vi "oa_Build Spectral Info for Order Magnitude and Phase (N Channels).vi"(0 "channel info":T8[](array[typedef]) {"channel info"."pregain" format="%.2f"; "channel info"."weighting filter" items=["Linear", "A-weighting", "B-weighting", "C-weighting", "ITU-R 468-4", "Dolby", "CCITT", "C-message", "Wb", "Wc", "Wd", "We", "Wf", "Wh", "Wj", "Wk", "Wm", "AES17 20 kHz lowpass", "AES17 40 kHz lowpass", "AES17 20 kHz highpass", "AES17 40 kHz highpass"]; "channel info"."dB reference" format="%^.1e"; "channel info"."engineering units" items=["custom..."=0, "V"=1, "A"=21, "C"=30, "pC"=31, "s"=32, "-"=29, "Pa"=2, "N"=20, "g"=3, "m/s^2"=4, "m/s"=5, "m"=6, "mm/s"=12, "mm"=13, "micron/s"=14, "micron"=15, "in/s^2"=7, "in/s"=8, "in"=9, "mil/s"=10, "mil"=11, "rad/s^2"=16, "rad/s"=17, "rad"=18, "deg/s^2"=26, "deg/s"=27, "deg"=28, "RPM"=22, "cycle/s^2"=23, "Hz"=24, "cycle"=25, "strain"=19]; "channel info"."sensor sensitivity" format="%#_5f"}, 1 "reset? (T)":bool=TRUE, 5 "X axis selection":u16(ring)=2 items=["Time", "Revolution", "RPM"], 7 "unit labels":string[](array[string]), 9 "orders to compute":dbl[](array[numeric]) format="%.2f", 11 "error in (no error)":errorcluster, 12 "view":T1={"dB on? (T)"=FALSE, "unwrap phase? (T)"=TRUE, "unit in degree? (T)"=TRUE}) -> (4 "spectrum info":T2[](array[typedef]) {"x-axis units" items=["Time (s)"=0, "Frequency-CB (Hz)"=1, "Frequency-CPB (Hz)"=1248, "Frequency-Arbitrary (Hz)"=2357, "Quefrency (s)"=2, "Revolutions (rev)"=3, "Order"=4, "Speed (RPM)"=11, "Speed (rad/s)"=21, "Index"=65535]; "weighting filter" items=["Linear", "A-weighting", "B-weighting", "C-weighting", "ITU-R 468-4", "Dolby", "CCITT", "C-message", "Wb", "Wc", "Wd", "We", "Wf", "Wh", "Wj", "Wk", "Wm", "AES17 20 kHz lowpass", "AES17 40 kHz lowpass", "AES17 20 kHz highpass", "AES17 40 kHz highpass"]; "dB reference [EU]" format="%.2f"; "engineering units" items=["custom..."=0, "V"=1, "A"=21, "C"=30, "pC"=31, "s"=32, "-"=29, "Pa"=2, "N"=20, "g"=3, "m/s^2"=4, "m/s"=5, "m"=6, "mm/s"=12, "mm"=13, "micron/s"=14, "micron"=15, "in/s^2"=7, "in/s"=8, "in"=9, "mil/s"=10, "mil"=11, "rad/s^2"=16, "rad/s"=17, "rad"=18, "deg/s^2"=26, "deg/s"=27, "deg"=28, "RPM"=22, "cycle/s^2"=23, "Hz"=24, "cycle"=25, "strain"=19]; "spectral info"."window" items=["None "=0, "Hanning"=1, "Hamming"=2, "Blackman-Harris"=3, "Exact Blackman"=4, "Blackman"=5, "Flat Top"=6, "4 Term B-Harris "=7, "7 Term B-Harris"=8, "Low Sidelobe"=9, "Force - Exponential"=10, "Gaussian"=62]}, 15 "error out":errorcluster)   [LabVIEW 2017, in "SoundVib_Resampling.lvlib"]
uses:
  <vilib>/addons/Sound and Vibration/Order Analysis/Resample Order Tracking/SoundVib_Resampling.lvlib
  <vilib>/addons/_NISVFA/_Shared subVIs/Controls/svc_Resampled Channel Info.ctl
  <vilib>/addons/_NISVFA/_Shared subVIs/Controls/svc_Channel Info.ctl
  <vilib>/addons/_NISVFA/_Shared subVIs/Controls/svc_Engineering Units Text Ring.ctl
  <vilib>/addons/_NISVFA/_Shared subVIs/Controls/svc_Weighting Filter Text Ring.ctl
  <vilib>/addons/_NISVFA/_Shared subVIs/Controls/svc_Spectrum Info.ctl
  <vilib>/addons/_NISVFA/_Shared subVIs/Controls/svc_X-Axis Units.ctl
  <vilib>/addons/_NISVFA/_Shared subVIs/Controls/svc_Spectrum Type.ctl
  <vilib>/addons/_NISVFA/_Shared subVIs/Controls/svc_Complimentary Spectrum Units.ctl
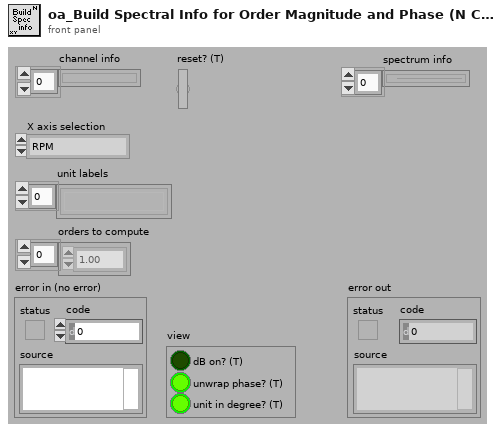
[diagram p1: front panel]
types:
  T1 = cluster{"dB on? (T)":bool, "unwrap phase? (T)":bool, "unit in degree? (T)":bool}
  T2 = typedef "svc_Spectrum Info.ctl" = cluster{"channel name":string, "description":string, "x-axis units":T3, "spectral info":cluster{"spectrum type":T4, "linear/dB":enum16{"linear", "dB"}, "window":u16, "window size":i32, "FFT size":i32}, "engineering units":T5, "custom label":string, "dB reference [EU]":dbl, "peak units":enum16{"rms", "peak", "peak-peak"}, "weighting filter":T6, "spectral density?":bool, "unit label":string, "spectrum skewed?":bool, "complimentary spectrum units":T7}
  T3 = typedef "svc_X-Axis Units.ctl" = u16
  T4 = typedef "svc_Spectrum Type.ctl" = enum16{"FFT Spectrum [complex]", "Amplitude [Magnitude]", "Power [Magnitude^2]", "Cross Spectrum [complex]", "Frequency Response [Complex]"}
  T5 = typedef "svc_Engineering Units Text Ring.ctl" = u16
  T6 = typedef "svc_Weighting Filter Text Ring.ctl" = u16
  T7 = typedef "svc_Complimentary Spectrum Units.ctl" = enum16{"none", "radians", "degrees", "cycles", "imaginary"}
  T8 = typedef "svc_Resampled Channel Info.ctl" = cluster{"channel name":string, "description":string, " channel info":T9}
  T9 = typedef "svc_Channel Info.ctl" = cluster{"sensor sensitivity":dbl, "engineering units":T5, "dB reference":dbl, "custom label":string, "weighting filter":T6, "pregain":dbl}
  T10 = cluster{"spectrum type":T4, "linear/dB":enum16{"linear", "dB"}, "window":u16, "window size":i32, "FFT size":i32}
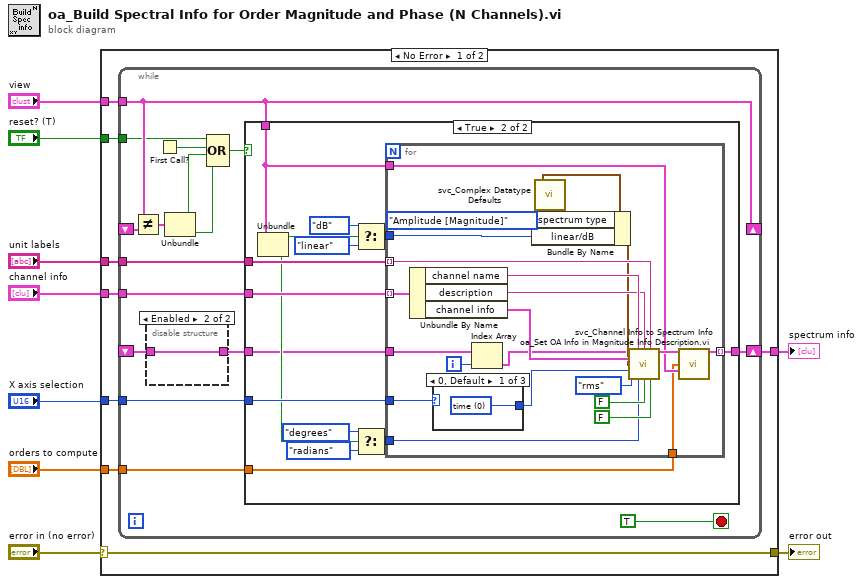
[diagram p0: block diagram]
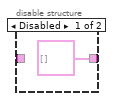
[diagram p2: hidden frame]
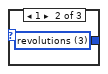
[diagram p4: hidden frame]
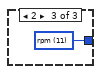
[diagram p5: hidden frame]
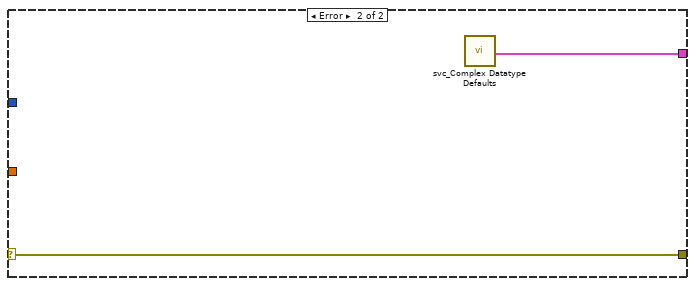
[diagram p6: hidden frame]
diagram:
  n1 = case shown="No Error" "error in (no error)" {
    selector: "error in (no error)" -> [w16 w78]
    tunnel: [w16 w78] -> w8
    tunnel: [w15 w77] -> w4
    tunnel: "channel info" -> [w17 _]
    tunnel: "unit labels" -> [w14 _]
    tunnel: "X axis selection" -> [w13 _]
    tunnel: "view" -> [w12 _]
    tunnel: "reset? (T)" -> [w11 _]
    tunnel: "orders to compute" -> [w10 _]
    frame No Error {
      n2 = while {
        tunnel: w17 -> [w33]
        tunnel: w14 -> [w31]
        tunnel: w13 -> [w30]
        shift-right: [w27] -> _
        shift-left: _ -> [w28]
        shift-right: [w32] -> w15
        shift-left: _ -> [w18]
        tunnel: w12 -> [w27]
        tunnel: w11 -> [w26]
        tunnel: w10 -> [w20]
        stop <- TRUE stop-if-true
        n3 = Not Equal?(x=w27, y=w28) -> (x != y?=w24:T1)
        n4 = disable-structure shown="Enabled" {
          disable-tunnel: [T2[] [] w35] -> w19
          disable-tunnel: w18 -> [_ w35]
          frame Disabled {
          }
          frame Enabled {
          }
        }
        n5 = First Call?() -> (First Call?: T/F=w25:bool)
        n6 = Unbundle(w24) -> ("dB on? (T)"=w23:bool, "unit in degree? (T)"=w22:bool)  [unwired: 1 out]
        n7 = Compound Arithmetic op=OR(w26, w25, w23, w22) -> (w21:bool)
        n8 = case shown="True" w21 {
          tunnel: w33 -> [_ w51]
          tunnel: [w36 w50] -> w32
          tunnel: w31 -> [_ w49]
          tunnel: w30 -> [_ w48]
          tunnel: w19 -> [w36 w39]
          tunnel: w27 -> [_ w38]
          tunnel: w20 -> [_ w37]
          frame False {
          }
          frame True {
            n9 = Unbundle(w38) -> ("dB on? (T)"=w44:bool, "unit in degree? (T)"=w43:bool)  [unwired: 1 out]
            n10 = Select(t=enum16{"linear", "dB"}."dB" ("spectral info.linear/dB"), s=w44, f=enum16{"linear", "dB"}."linear" ("spectral info.linear/dB")) -> (s? t:f=w45:enum16{"linear", "dB"})
            n11 = Select(t=svc_Complimentary_Spectrum_Units."degrees" ("complimentary spectrum units"), s=w43, f=svc_Complimentary_Spectrum_Units."radians" ("complimentary spectrum units")) -> (s? t:f=w40:T7)
            n12 = for {
              tunnel: w51 -> [w69] mode=indexing
              tunnel: [w54] -> w50 mode=indexing
              tunnel: w49 -> [w67] mode=indexing
              tunnel: w48 -> [w68]
              tunnel: w45 -> [w59]
              tunnel: w40 -> [w63]
              tunnel: w39 -> [w58]
              tunnel: w38 -> [w53]
              tunnel: w37 -> [w52]
              i -> [w57]
              n13 = Unbundle By Name(w69) -> ("channel name"=w73:string, "description"=w72:string, "channel info"=w66:T9)
              n14 = case shown="0, Default" w68 {
                tunnel: [w74 w75 w76] -> w64
                frame 0, Default {
                  w74 = u16 0 items=["time"=0, "frequency"=1, "quefrency"=2, "revolutions"=3, "order"=4, "rpm"=11] ("x-axis units")
                }
                frame 1 {
                  w75 = u16 3 items=["time"=0, "frequency"=1, "quefrency"=2, "revolutions"=3, "order"=4, "rpm"=11] ("x-axis units")
                }
                frame 2 {
                  w76 = u16 11 items=["time"=0, "frequency"=1, "quefrency"=2, "revolutions"=3, "order"=4, "rpm"=11] ("x-axis units")
                }
              }
              n15 = Index Array(array=w58, index=w57) -> (element=w56:T2)
              n16 = call <vilib>:"svc_Complex Datatype Defaults.vi"() -> ("spectral info"=w62:T10)  [unwired: 11 in, 8 out]
              n17 = Bundle By Name(cluster=w62, "spectrum type"=svc_Spectrum_Type."Amplitude [Magnitude]", "linear/dB"=w59) -> (w61:T10)
              n18 = call <vilib>:"svc_Channel Info to Spectrum Info.vi"("spectrum info in"=w56, "channel name"=w73, "description"=w72, "unit label"=w67, "channel info"=w66, "spectral info"=w61, "x-axis units"=w64, "peak units"=enum16{"rms", "peak", "peak-peak"}."rms", "complimentary spectrum units"=w63, "spectral density?"=FALSE, "spectrum skewed?"=FALSE) -> ("spectrum info out"=w55:T2)  [unwired: 4 in]
              n19 = call <vilib>:"oa_Set OA Info in Magnitude Info Description.vi.vi"("magnitude info"=w55, "orders to compute"=w52, "view"=w53) -> ("magnitude info out"=w54:T2)  [unwired: 11 in, 1 out]
            }
          }
        }
      }
    }
    frame Error {
      n20 = call <vilib>:"svc_Complex Datatype Defaults.vi"() -> ("empty array of spectrum info"=w77:T2[])  [unwired: 11 in, 8 out]
    }
  }
  "error out" <- w8
  "spectrum info" <- w4
